vi "Switch Output Channel.vi"(8 "error in (no error)":errorcluster, 9 "New Channel":u8, 10 "Old Channel":u8, 11 "class data in":refnum<class "CS Emulation.lvclass">) -> (0 "error out":errorcluster, 3 "class data out":refnum<class "CS Emulation.lvclass">)   [LabVIEW 2013, in "CS Emulation.lvclass"]
uses:
  Lib.llb/CS Emulation.lvclass
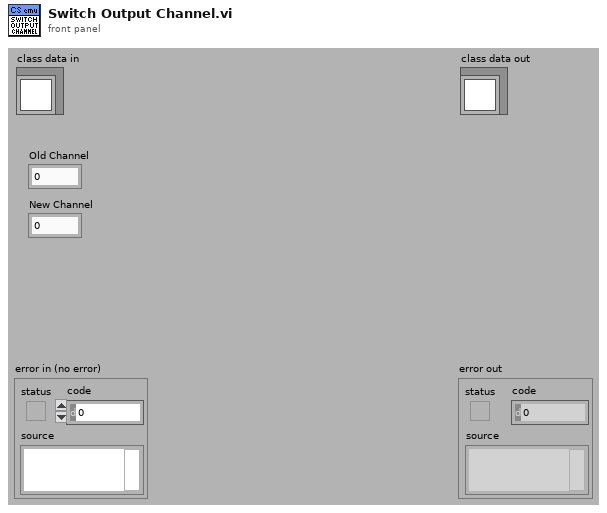
[diagram p1: front panel]
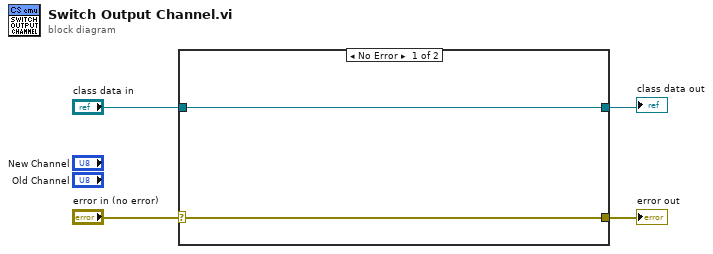
[diagram p0: block diagram]
diagram:
  n1 = case shown="No Error" "error in (no error)" {
    selector: "error in (no error)" -> [w6 w8]
    tunnel: [w6 w8] -> w3
    tunnel: "class data in" -> [w5 w7]
    tunnel: [w5 w7] -> w1
    frame No Error {
    }
    frame Error {
    }
  }
  "error out" <- w3
  "class data out" <- w1
